vi "Create Master Instance (Serial copy).vi"(7 "unit ID":u8=1, 8 "error in (no error)":errorcluster, 11 "serial master instance copy":refnum<class "Modbus Master.lvclass">) -> (0 "error out":errorcluster, 3 "serial master instance":refnum<class "Modbus Master.lvclass">)   [LabVIEW 2021, in "API Main.lvlib"]
doc: "Creates a serial or TCP Modbus master instance. You must manually select the polymorphic instance to use."
uses:
  API Main.lvlib
  Master/Modbus Master.lvclass
  Master/Modbus Master.lvclass/Modbus Master.ctl
  Network Protocol/Network Master/Network Master.lvclass/Network Master.ctl
  Transmission Data Unit/Transmission Data Unit.lvclass/Transmission Data Unit.ctl
  Transmission Data Unit/Transmission Data Unit.lvclass
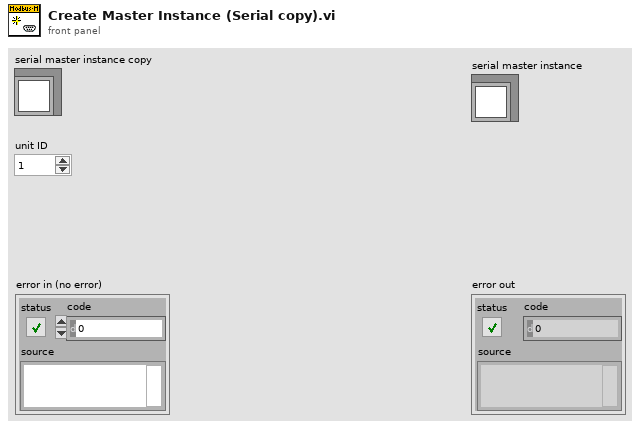
[diagram p1: front panel]
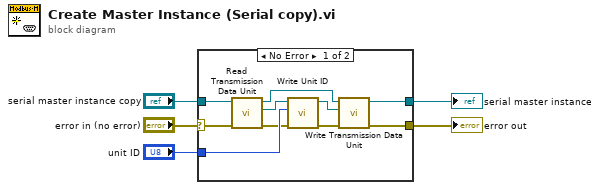
[diagram p0: block diagram]
diagram:
  n1 = case shown="No Error" "error in (no error)" {
    selector: "error in (no error)" -> [w14 w16]
    tunnel: [w7 w16] -> w5
    tunnel: [w6 _] -> w4
    tunnel: "unit ID" -> [w13 _]
    tunnel: "serial master instance copy" -> [w15 _]
    frame No Error {
      n2 = call "Read Transmission Data Unit.vi"("error in"=w14, "Modbus instance in"=w15) -> ("error out"=w11:errorcluster, "transmission data unit"=w12:refnum<class "Transmission Data Unit.lvclass">, "Modbus instance out"=w8:refnum<class "Modbus Master.lvclass">)  [unwired: 7 in]
      n3 = call "Write Unit ID.vi"("error in"=w11, "unit ID"=w13, "transmission data unit in"=w12) -> ("error out"=w10:errorcluster, "transmission data unit out"=w9:refnum<class "Transmission Data Unit.lvclass">)  [unwired: 7 in]
      n4 = call "Write Transmission Data Unit.vi"("error in"=w10, "transmission data unit"=w9, "Modbus instance in"=w8) -> ("error out"=w7:errorcluster, "Modbus instance out"=w6:refnum<class "Modbus Master.lvclass">)  [unwired: 7 in]
    }
    frame Error {
    }
  }
  "error out" <- w5
  "serial master instance" <- w4
